vi "Async.Engine.Close.vi"(8 "error in":errorcluster, 11 "Async in":refnum<class "VS Plugin Inline Async API.lvclass">=refnum) -> (0 "error out":errorcluster, 3 "Async out":refnum<class "VS Plugin Inline Async API.lvclass">)   [LabVIEW 2023, in "VS Plugin Inline Async API.lvlib" / "VS Plugin Inline Async API.lvclass"]
uses:
  VS Plugin Inline Async API.lvclass
  VS Plugin Inline Async API.lvclass/VS Plugin Inline Async API.ctl
  _Plugin Data Access Engine/Plugin Data Access Engine/Plugin Data Access Engine.lvclass
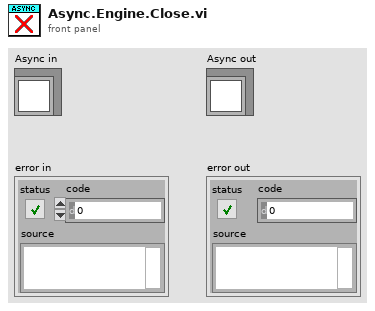
[diagram p1: front panel]
types:
  T1 = typedef "VS Plugin Inline Async API.lvlib/VS Plugin Inline Async API.lvclass/Error Handling Settings.ctl" = cluster{"Write to SystemLog (F)":bool}
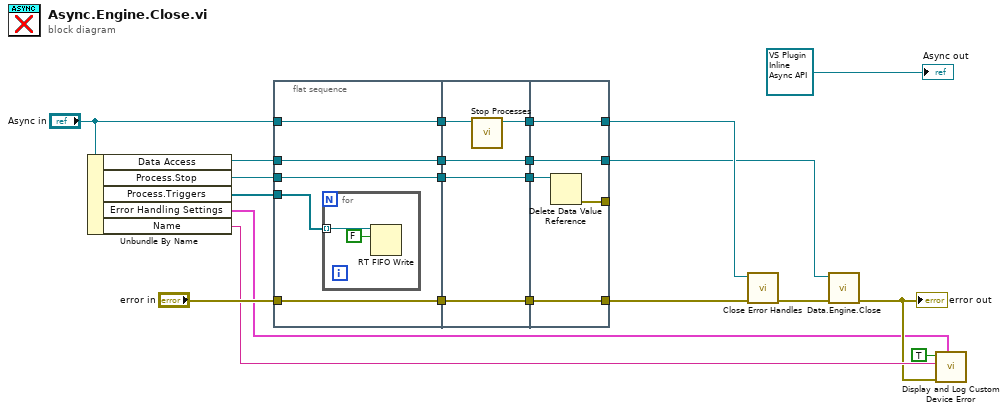
[diagram p0: block diagram]
diagram:
  n1 = Unbundle By Name("Async in") -> ("Data Access"=w7:refnum<class "Plugin Data Access Engine.lvclass">, "Process.Stop"=w15:refnum<data-value>, "Process.Triggers"=w6:refnum<k33>[], "Error Handling Settings"=w1:T1, "Name"=w17:string)
  n2 = flat-sequence {
    tunnel: [w27] -> w22
    tunnel: "error in" -> [w27]
    tunnel: [w26] -> w16
    tunnel: "Async in" -> [w26]
    tunnel: w15 -> [w25]
    tunnel: [w25] -> w14
    tunnel: [w24] -> w8
    tunnel: w7 -> [w24]
    tunnel: w6 -> [w23]
    tunnel: [w34] -> w5
    tunnel: w22 -> [w34]
    tunnel: w16 -> [w33]
    tunnel: [w32] -> w4
    tunnel: w14 -> [w32]
    tunnel: [w31] -> w3
    tunnel: [w30] -> w2
    tunnel: w8 -> [w30]
    tunnel: [w39] -> w20
    tunnel: w5 -> [w39]
    tunnel: w4 -> [w38]
    tunnel: [w37] -> w12
    tunnel: w3 -> [w37]
    tunnel: [w36] -> _
    tunnel: [w35] -> w9
    tunnel: w2 -> [w35]
    frame #0 {
      n3 = for {
        tunnel: w23 -> [w29] mode=indexing
        n4 = RT FIFO Write(0:w29, 1:FALSE ("element")) -> ()  [unwired: 3 in, 4 out]
      }
    }
    frame #1 {
      n5 = call "Stop Processes.vi"("VS Plugin Inline Async API in"=w33) -> ("VS Plugin Inline Async API out"=w31:refnum<class "VS Plugin Inline Async API.lvclass">)  [unwired: 10 in]
    }
    frame #2 {
      n6 = Delete Data Value Reference(data value reference=w38) -> (error out=w36:errorcluster)  [unwired: 1 in, 1 out]
    }
  }
  n7 = call "Close Error Handles.vi"("error in"=w20, "Async in"=w12) -> ("error out"=w11:errorcluster)  [unwired: 8 in, 1 out]
  n8 = call "Data.Engine.Close.vi"("error in"=w11, "Data Access API in"=w9) -> ("error out"=w10:errorcluster)  [unwired: 8 in, 1 out]
  "error out" <- w10
  n9 = call "Display and Log Custom Device Error.vi"("Error Log Settings"=w1, "error out"=w10, "Your code's public name"=w17, "Custom Device? (T)"=TRUE) -> ()  [unwired: 8 in]
  "Async out" <- refnum<class "VS Plugin Inline Async API.lvclass"> refnum ("Async out")
